vi "UpdateXml.vi"(8 "error in (no error)":errorcluster, 11 "Library Builder in":refnum<class "Library Builder.lvclass">) -> (0 "error out":errorcluster, 3 "Library Builder out":refnum<class "Library Builder.lvclass">)   [LabVIEW 2020, in "Library Builder.lvclass"]
uses:
  Library Builder.lvclass
  Library Builder.lvclass/Library Builder.ctl
  Shared/Shared.lvlib
panel:
  out "XML Path":path
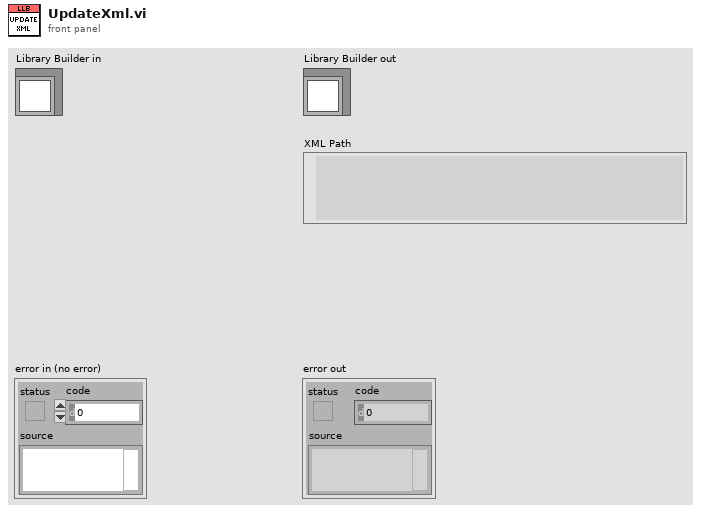
[diagram p1: front panel]
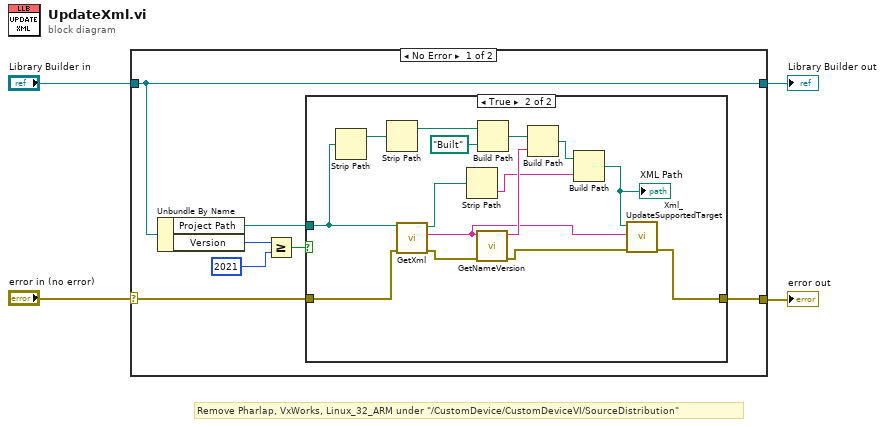
[diagram p0: block diagram]
diagram:
  # "Remove Pharlap, VxWorks, Linux_32_ARM under \"/CustomDevice/CustomDeviceVI/SourceDistribution\""
  n1 = case shown="No Error" "error in (no error)" {
    selector: "error in (no error)" -> [w10 w29]
    tunnel: [w7 w29] -> w3
    tunnel: [w11 w28] -> w1
    tunnel: "Library Builder in" -> [w11 w28]
    frame No Error {
      n2 = Unbundle By Name(w11) -> ("Project Path"=w6:path, "Version"=w8:u32)
      n3 = Greater Or Equal?(x=w8, y=u32 2021 ("Version")) -> (x >= y?=w5:bool)
      n4 = case shown="True" w5 {
        tunnel: w10 -> [w12 w27]
        tunnel: w6 -> [_ w22]
        tunnel: [w12 w14] -> w7
        frame False {
        }
        frame True {
          n5 = Strip Path(path=w22) -> (stripped path=w25:path)  [unwired: 1 out]
          n6 = Strip Path(path=w25) -> (stripped path=w24:path)  [unwired: 1 out]
          n7 = call "GetXml.vi"("error in (no error)"=w27, "Project Path"=w22) -> ("error out"=w26:errorcluster, "XML String"=w15:string, "XML Path"=w18:path)  [unwired: 7 in]
          n8 = Strip Path(path=w18) -> (name=w13:string)  [unwired: 1 out]
          n9 = call "GetNameVersion.vi"("error in (no error)"=w26, "XML String"=w15) -> ("error out"=w19:errorcluster, "Custom Device Name"=w20:string)  [unwired: 7 in, 1 out]
          n10 = Build Path(base path=w24, name or relative path=path "Built") -> (appended path=w21:path)
          n11 = Build Path(base path=w21, name or relative path=w20) -> (appended path=w17:path)
          n12 = Build Path(base path=w17, name or relative path=w13) -> (appended path=w16:path)
          "XML Path" <- w16
          n13 = call "Xml_UpdateSupportedTarget.vi"("error in (no error)"=w19, "XML String"=w15, "XML Path"=w16) -> ("error out"=w14:errorcluster)  [unwired: 8 in]
        }
      }
    }
    frame Error {
    }
  }
  "error out" <- w3
  "Library Builder out" <- w1
